vi "_Update N Graph.vi"(4 "TIC (F)":bool, 5 "Auto Scale":bool, 6 "Graph Ref":refnum<vi>, 7 "Array":T2[](array[typedef]), 8 "error in (no error)":errorcluster, 9 "Log Scale":bool, 10 "CPS":bool, 11 "Averaging":bool) -> (3 "Graph Property":T1)   [LabVIEW 2015]
uses:
  Type/_Data.ctl
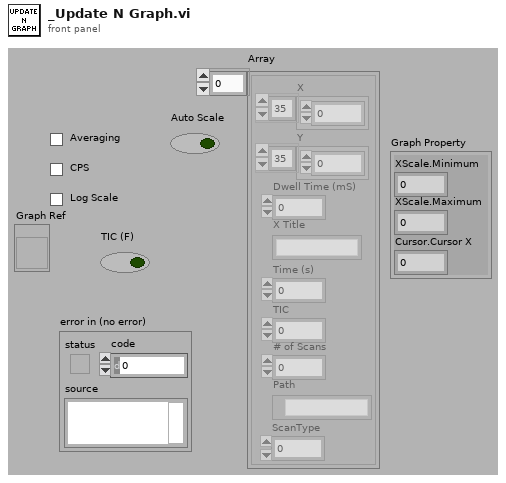
[diagram p1: front panel]
types:
  T1 = cluster{"XScale.Minimum":dbl, "XScale.Maximum":dbl, "Cursor.Cursor X":dbl}
  T2 = typedef "_Data.ctl" = cluster{"X":dbl[], "Y":dbl[], "Dwell Time (mS)":dbl, "X Title":string, "Time (s)":dbl, "TIC":u32, "# of Scans":i32, "Path":path, "ScanType":i32}
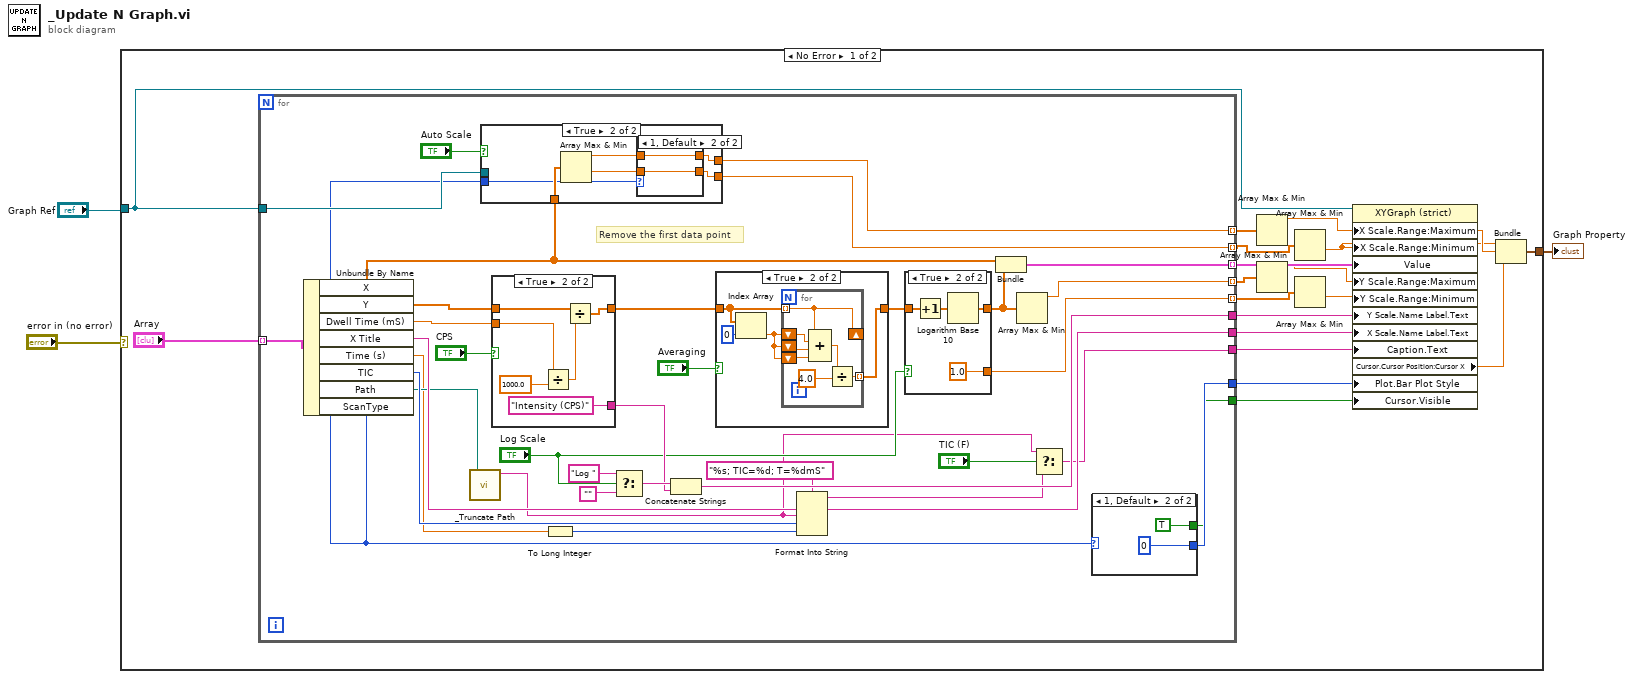
[diagram p0: block diagram]
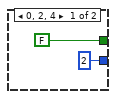
[diagram p2: hidden frame]
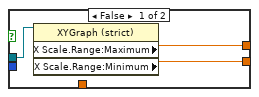
[diagram p3: hidden frame]
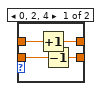
[diagram p4: hidden frame]
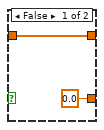
[diagram p5: hidden frame]
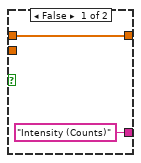
[diagram p7: hidden frame]
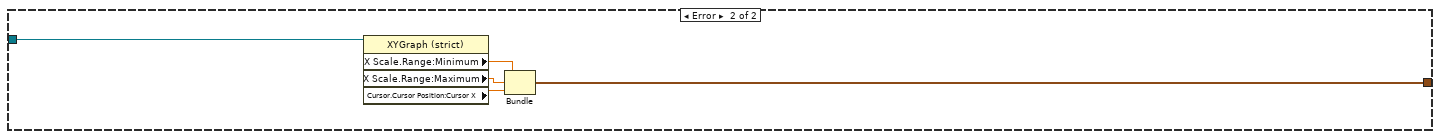
[diagram p8: hidden frame]
diagram:
  n1 = case shown="No Error" "error in (no error)" {
    tunnel: [w16 w103] -> w2
    tunnel: "Graph Ref" -> [w14 w106]
    frame No Error {
      n2 = for {
        tunnel: "Array" -> [w47] mode=indexing
        tunnel: [w45] -> w20 mode=indexing
        tunnel: [w44] -> w19
        tunnel: [w43] -> w18
        tunnel: [w39] -> w9 mode=indexing
        tunnel: [w38] -> w17 mode=indexing
        tunnel: [w37] -> w5 mode=indexing
        tunnel: [w36] -> w7 mode=indexing
        tunnel: w14 -> [w34]
        tunnel: [w29] -> w13
        tunnel: [w26] -> w12
        tunnel: [w23] -> w11
        # "Remove the first data point"
        n3 = Unbundle By Name(w47) -> ("X"=w30:dbl[], "Y"=w27:dbl[], "Dwell Time (mS)"=w46:dbl, "X Title"=w43:string, "Time (s)"=w33:dbl, "TIC"=w42:u32, "Path"=w40:path, "ScanType"=w28:i32)
        n4 = call "_Truncate Path.vi"("Path"=w40) -> ("String"=w22:string)  [unwired: 1 in, 5 out]
        n5 = case shown="True" "Auto Scale" {
          tunnel: w30 -> [_ w69]
          tunnel: [w62 w64] -> w39
          tunnel: [w63 w65] -> w38
          tunnel: w34 -> [w61 _]
          tunnel: w28 -> [_ w68]
          frame False {
            n6 = property class="XYGraph (strict)"(reference=w61) -> ("X Scale.Range:Maximum"=w63:dbl, "X Scale.Range:Minimum"=w62:dbl)  [unwired: 1 in, 2 out]
          }
          frame True {
            n7 = Array Max & Min(array=w69) -> (max value=w67:dbl, min value=w66:dbl)  [unwired: 2 out]
            n8 = case shown="1, Default" w68 {
              tunnel: w67 -> [w73 w75]
              tunnel: w66 -> [w71 w74]
              tunnel: [w72 w75] -> w65
              tunnel: [w70 w74] -> w64
              frame 0, 2, 4 {
                n9 = Increment(x=w73) -> (x+1=w72:dbl)
                n10 = Decrement(x=w71) -> (x-1=w70:dbl)
              }
              frame 1, Default {
              }
            }
          }
        }
        n11 = case shown="True" "CPS" {
          tunnel: w27 -> [w95 w100]
          tunnel: [w95 w98] -> w31
          tunnel: ["Intensity (Counts)" "Intensity (CPS)"] -> w51
          tunnel: w46 -> [_ w96]
          frame False {
          }
          frame True {
            n12 = Divide(x=w96, y=1000.0) -> (x/y=w99:dbl)
            n13 = Divide(x=w100, y=w99) -> (x/y=w98:dbl[])
          }
        }
        n14 = To Long Integer(number=w33) -> (32bit integer=w32:i32)
        n15 = Select(t="Log ", s="Log Scale", f="") -> (s? t:f=w52:string)
        n16 = Concatenate Strings(w52, w51) -> (w44:string)
        n17 = case shown="True" "Averaging" {
          tunnel: w31 -> [w82 w84]
          tunnel: [w82 w83] -> w50
          frame False {
          }
          frame True {
            n18 = Index Array(array=w84, index=0) -> (element=w85:dbl)
            n19 = for {
              shift-right: [w90] -> _
              shift-left: w85 -> [w93]
              shift-left: w85 -> [w92]
              shift-left: w85 -> [w91]
              tunnel: w84 -> [w90] mode=indexing
              tunnel: [w87] -> w83 mode=indexing
              n20 = Compound Arithmetic op=ADD(w90, w93, w92, w91) -> (w89:dbl)
              n21 = Divide(x=w89, y=4.0) -> (x/y=w87:dbl)
            }
          }
        }
        n22 = Format Into String(format string="%s; TIC=%d; T=%dmS", w22, w42, w32) -> (resulting string=w24:string)  [unwired: 2 in, 1 out]
        n23 = case shown="True" "Log Scale" {
          tunnel: w50 -> [w77 w81]
          tunnel: [w77 w80] -> w49
          tunnel: [0.0 ("y") 1.0 ("y")] -> w37
          frame False {
          }
          frame True {
            n24 = Increment(x=w81) -> (x+1=w78:dbl[])
            n25 = Logarithm Base 10(1:w78) -> (0:w80:dbl[])
          }
        }
        n26 = Bundle("X"=w30, "Y"=w49) -> (w45:cluster{"X":dbl[], "Y":dbl[]})  [unwired: 1 out]
        n27 = Array Max & Min(array=w49) -> (max value=w36:dbl)  [unwired: 3 out]
        n28 = Select(t=w22, s="TIC (F)", f=w24) -> (s? t:f=w23:string)
        n29 = case shown="1, Default" w28 {
          tunnel: [u8 2 ("Plot.Bar Plot Style") u8 0 ("Plot.Bar Plot Style")] -> w29
          tunnel: [FALSE TRUE] -> w26
          frame 0, 2, 4 {
          }
          frame 1, Default {
          }
        }
      }
      n30 = Array Max & Min(array=w17) -> (max value=w10:dbl)  [unwired: 3 out]
      n31 = Array Max & Min(array=w7) -> (max value=w6:dbl)  [unwired: 3 out]
      n32 = Array Max & Min(array=w9) -> (min value=w8:dbl)  [unwired: 3 out]
      n33 = Array Max & Min(array=w5) -> (min value=w4:dbl)  [unwired: 3 out]
      n34 = property class="XYGraph (strict)"(reference=w14, "X Scale.Range:Maximum"=w10, "X Scale.Range:Minimum"=w8, "Value"=w20, "Y Scale.Range:Maximum"=w6, "Y Scale.Range:Minimum"=w4, "Y Scale.Name Label.Text"=w19, "X Scale.Name Label.Text"=w18, "Caption.Text"=w11, "Plot.Bar Plot Style"=w13, "Cursor.Visible"=w12) -> ("Cursor.Cursor Position:Cursor X"=w15:dbl)  [unwired: 1 in, 2 out]
      n35 = Bundle(w8, w10, "Cursor.Cursor X"=w15) -> (w16:cluster{dbl, dbl, "Cursor.Cursor X":dbl})  [unwired: 1 out]
    }
    frame Error {
      n36 = property class="XYGraph (strict)"(reference=w106) -> ("X Scale.Range:Minimum"=w105:dbl, "X Scale.Range:Maximum"=w104:dbl, "Cursor.Cursor Position:Cursor X"=w102:dbl)  [unwired: 1 in, 2 out]
      n37 = Bundle("XScale.Minimum"=w105, "XScale.Maximum"=w104, "Cursor.Cursor X"=w102) -> (w103:T1)  [unwired: 1 out]
    }
  }
  "Graph Property" <- w2
